vi "Update Destinations Count.vi"(8 "error in (no error)":errorcluster, 11 "BuildSpec in":refnum<vi>) -> (0 "error out":errorcluster, 3 "BuildSpec out":refnum<vi>)   [LabVIEW 2019, in "Project Sync Tools.lvclass"]
uses:
  Project Sync Tools.lvclass
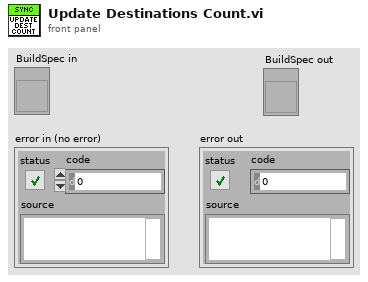
[diagram p1: front panel]
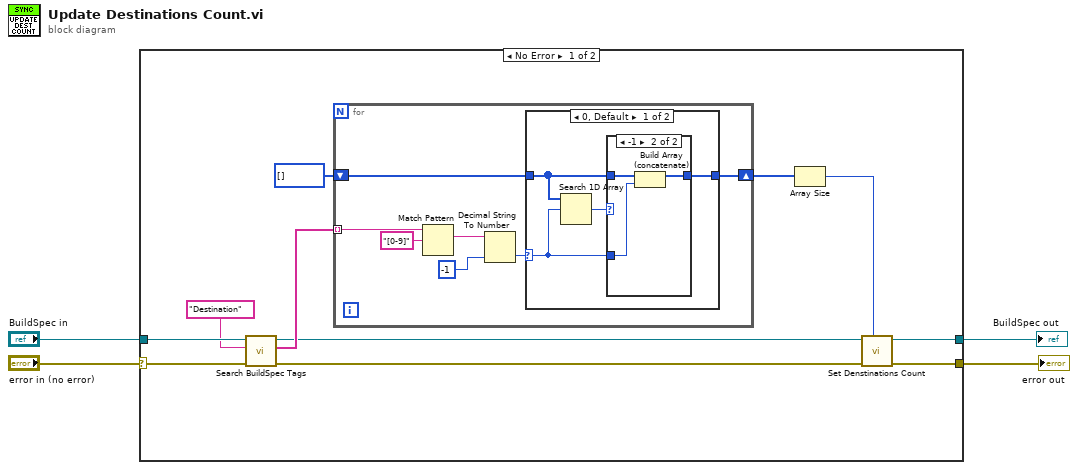
[diagram p0: block diagram]
diagram:
  n1 = case shown="No Error" "error in (no error)" {
    selector: "error in (no error)" -> [w5 w32]
    tunnel: "BuildSpec in" -> [w15 w33]
    tunnel: [w9 w32] -> w3
    tunnel: [w6 w33] -> w2
    frame No Error {
      n2 = call "Search BuildSpec Tags.vi"("error in (no error)"=w5, "Regular expression"="Destination", "BuildSpec in"=w15) -> ("error out"=w10:errorcluster, "Tag Names"=w12:string[], "BuildSpec out"=w8:refnum<vi>)  [unwired: 6 in]
      n3 = for {
        tunnel: w12 -> [w22] mode=indexing
        shift-right: [w17] -> w14
        shift-left: i32[] [] -> [w18]
        n4 = Match Pattern(string=w22, regular expression="[0-9]") -> (match substring=w20:string)  [unwired: 1 in, 3 out]
        n5 = Decimal String To Number(string=w20, default (0L)=-1 ("default (0 I32)")) -> (number=w16:i32)  [unwired: 1 in, 1 out]
        n6 = case shown="0, Default" w16 {
          selector: w16 -> [w23 _]
          tunnel: w18 -> [w25 w31]
          tunnel: [w24 w31] -> w17
          frame 0, Default {
            n7 = Search 1D Array(1D array=w25, element=w23) -> (index of element=w26:i32)  [unwired: 1 in]
            n8 = case shown="-1" w26 {
              tunnel: w25 -> [w27 w30]
              tunnel: w23 -> [_ w29]
              tunnel: [w27 w28] -> w24
              frame 0, Default {
              }
              frame -1 {
                n9 = Build Array (concatenate)(w30, w29) -> (w28:i32[])
              }
            }
          }
          frame -1 {
          }
        }
      }
      n10 = Array Size(array=w14) -> (size(s)=w7:i32)
      n11 = call "Set Denstinations Count.vi"("Destination Count"=w7, "error in (no error)"=w10, "BuildSpect in"=w8) -> ("error out"=w9:errorcluster, "BuildSpec out"=w6:refnum<vi>)  [unwired: 7 in]
    }
    frame Error {
    }
  }
  "error out" <- w3
  "BuildSpec out" <- w2
